vi "draw.vi"() -> ()   [LabVIEW 2014]
uses:
  <vilib>/Analysis/1siggen.llb/Ramp Pattern by Samples.vi
  <vilib>/Analysis/NI_AALBase.lvlib
panel:
  out "XY Graph":T1(graph)
  in  "zero":bool
  in  "stop":bool
  in  "start":bool
  in  "amplitude_um":dbl
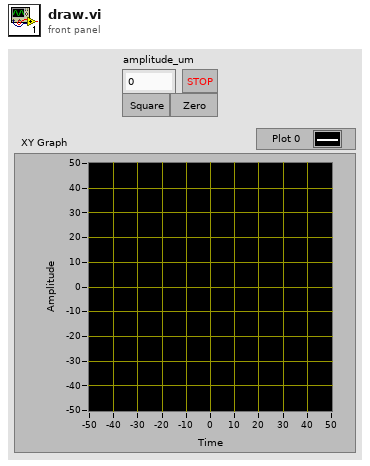
[diagram p1: front panel]
types:
  T1 = cluster{"Ramp Pattern":dbl[], "Ramp Pattern":dbl[]}
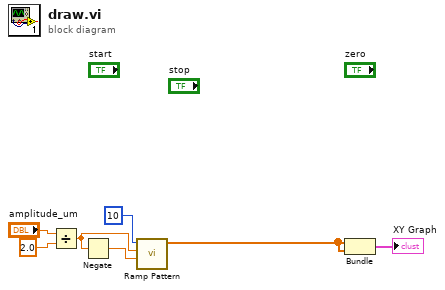
[diagram p0: block diagram]
diagram:
  n1 = Divide(x="amplitude_um", y=2.0) -> (x/y=w4:dbl)
  n2 = Negate(x=w4) -> (-x=w5:dbl)
  n3 = call-poly <vilib>:"Ramp Pattern.vi"("start"=w5, "end"=w4, "samples"=10) -> ("Ramp Pattern"=w2:dbl[])  [unwired: 7 in, 1 out]
  n4 = Bundle("Ramp Pattern"=w2, "Ramp Pattern"=w2) -> (→"XY Graph":T1)  [unwired: 1 in]
